vi "Launch Analog Input.vi"(8 "error in (no error)":errorcluster, 11 "Top in":refnum<class "Top.lvclass">) -> (0 "error out":errorcluster, 3 "Top out":refnum<class "Top.lvclass">)   [LabVIEW 2021, in "Top.lvlib" / "Top.lvclass"]
uses:
  Top.lvclass
  C:/Program Files/National Instruments/LabVIEW 2021/vi.lib/ActorFramework/Actor/Actor.lvclass
  <vilib>/NathanCo/Analog Tasks/Utilities/Analog Configuration Parameters.ctl
  Top.lvclass/Top.ctl
  <vilib>/NathanCo/Analog Tasks/Analog Input/Analog Input/Analog Input/Analog Input.lvclass
  <vilib>/ActorFramework/Actor/Actor.lvclass
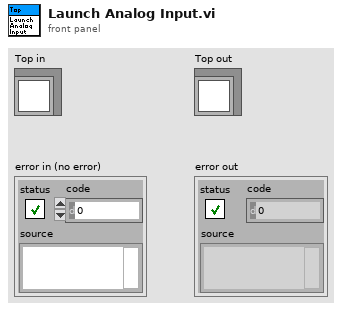
[diagram p1: front panel]
types:
  T1 = typedef "Analog Configuration Parameters.ctl" = cluster{"Terminal Configuration":i32, "Minimum Voltage":dbl, "Maximum Voltage":dbl, "Simulated?":bool, "Device":string, "Device Number":string, "Channel":string, "NI_ChannelName":string}
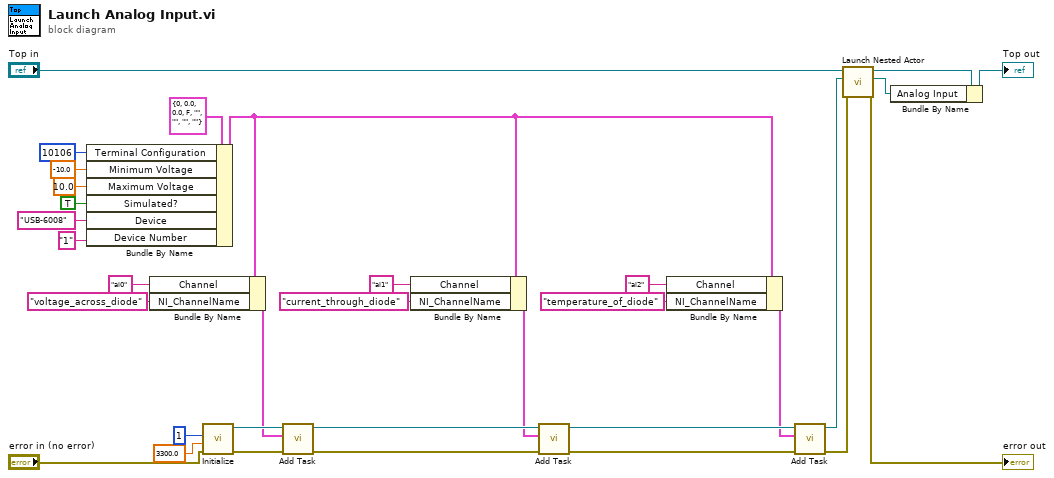
[diagram p0: block diagram]
diagram:
  n1 = Bundle By Name(cluster=T1 {"Terminal Configuration"=0, "Minimum Voltage"=0.0, "Maximum Voltage"=0.0, "Simulated?"=FALSE, "Device"="", "Device Number"="", "Channel"="", "NI_ChannelName"=""} ("Analog Configuration Parameters"), "Terminal Configuration"=10106, "Minimum Voltage"=-10.0, "Maximum Voltage"=10.0, "Simulated?"=TRUE, "Device"="USB-6008", "Device Number"="1") -> (w12:T1)
  n2 = Bundle By Name(cluster=w12, "Channel"="ai0", "NI_ChannelName"="voltage_across_diode") -> (w9:T1)
  n3 = call <vilib>:"Initialize.vi"("error in (no error)"="error in (no error)", "Rate"=3300.0, "Number Of Samples Per Channel"=1) -> ("error out"=w25:errorcluster, "Analog Input out"=w30:refnum<class "Analog Input.lvclass">)  [unwired: 7 in]
  n4 = call <vilib>:"Add Task.vi"("error in (no error)"=w25, "Analog Configuration Parameters"=w9, "Analog Input in"=w30) -> ("error out"=w26:errorcluster, "Analog Input out"=w29:refnum<class "Analog Input.lvclass">)  [unwired: 7 in]
  n5 = Bundle By Name(cluster=w12, "Channel"="ai1", "NI_ChannelName"="current_through_diode") -> (w10:T1)
  n6 = call <vilib>:"Add Task.vi"("error in (no error)"=w26, "Analog Configuration Parameters"=w10, "Analog Input in"=w29) -> ("error out"=w27:errorcluster, "Analog Input out"=w28:refnum<class "Analog Input.lvclass">)  [unwired: 7 in]
  n7 = Bundle By Name(cluster=w12, "Channel"="ai2", "NI_ChannelName"="temperature_of_diode") -> (w11:T1)
  n8 = call <vilib>:"Add Task.vi"("error in (no error)"=w27, "Analog Configuration Parameters"=w11, "Analog Input in"=w28) -> ("error out"=w23:errorcluster, "Analog Input out"=w31:refnum<class "Analog Input.lvclass">)  [unwired: 7 in]
  n9 = call <vilib>:"Launch Nested Actor.vi"("error in (no error)"=w23, "Nested Actor"=w31, "Caller Actor in"="Top in") -> ("error out"=→"error out":errorcluster, "Nested Actor's Enqueuer"=w1:refnum<class "Message Enqueuer.lvclass">, "Caller Actor out"=w32:refnum<class "Top.lvclass">)  [unwired: 6 in]
  n10 = Bundle By Name(cluster=w32, "Analog Input"=w1) -> (→"Top out":refnum<class "Top.lvclass">)
